vi "ScaleXAndRotateArray.vi"(1 "Scale":dbl=-1.0 format="%#_13g", 2 "Angle":dbl, 3 "X, Y, Z Input":dbl[](array[numeric])) -> (0 "c * X', Y', Z Output":dbl[](array[numeric]))   [LabVIEW 2017]
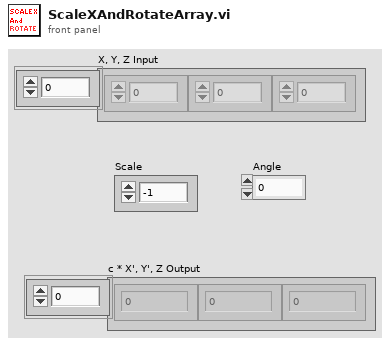
[diagram p1: front panel]
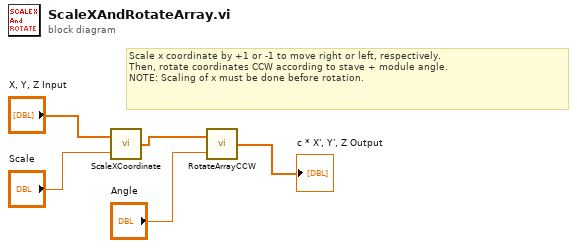
[diagram p0: block diagram]
diagram:
  # "Scale x coordinate by +1 or -1 to move right or left, respectively.\nThen, rotate coordinates CCW according to stave + module angle.\nNOTE: Scaling of x must be done before rotation."
  n1 = call "ScaleXCoordinate.vi"("Scale"="Scale", "X, Y, Z Input"="X, Y, Z Input") -> ("c * X, Y, Z Output"=w3:dbl[])
  n2 = call "RotateArrayCCW.vi"("Angle"="Angle", "X, Y, Z Input"=w3) -> ("X', Y', Z Output"=→"c * X', Y', Z Output":dbl[])  [unwired: 1 in]
